vi "PhotoEncoder.vi"(6 "Value":bool, 7 "Array":i16[](array[numeric]), 9 "Numeric 2":dbl, 10 "DigitalInputDevRef":T1, 11 "Numeric":dbl) -> ()   [LabVIEW 2015]
uses:
  <vilib>/Rock Robotics/WPI/DigitalInput/WPI_DigitalInputDevRef.ctl
  <vilib>/Rock Robotics/SystemInterfaces/DIO/FPGA_DIOChannel.ctl
  Wheel Gun Test/Robot Global Data.vi
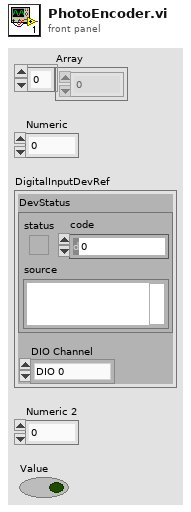
[diagram p1: front panel]
types:
  T1 = typedef "WPI_DigitalInputDevRef.ctl" = cluster{"DevStatus":errorcluster, "DIO Channel":T2}
  T2 = typedef "FPGA_DIOChannel.ctl" = enum8{"DIO 0", "DIO 1", "DIO 2", "DIO 3", "DIO 4", "DIO 5", "DIO 6", "DIO 7", "DIO 8", "DIO 9", "DIO MXP 0", "DIO MXP 1", "DIO MXP 2", "DIO MXP 3", "DIO MXP 4", "DIO MXP 5", "DIO MXP 6", "DIO MXP 7", "DIO MXP 8", "DIO MXP 9", "DIO MXP 10", "DIO MXP 11", "DIO MXP 12", "DIO MXP 13", "DIO MXP 14", "DIO MXP 15", "Invalid"}
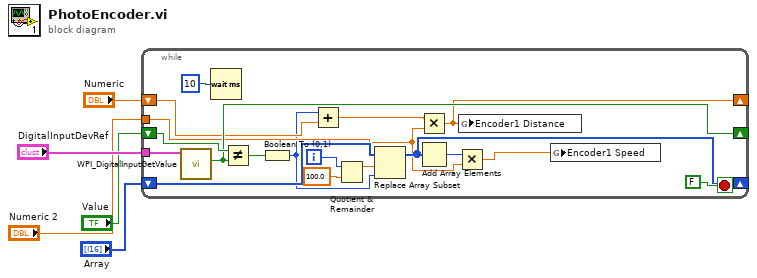
[diagram p0: block diagram]
diagram:
  n1 = while {
    shift-right: [w20] -> _
    shift-left: "Value" -> [w21]
    shift-right: [w8] -> _
    shift-left: "Numeric" -> [w19]
    shift-right: [w17] -> _
    shift-left: "Array" -> [w18]
    tunnel: "Numeric 2" -> [w14]
    tunnel: "DigitalInputDevRef" -> [w9]
    i -> [w12]
    stop <- FALSE stop-if-true
    n2 = call <vilib>:"WPI_DigitalInputGetValue.vi"("DigitalInputDevRef"=w9) -> ("Value"=w20:bool)  [unwired: 8 in, 2 out]
    n3 = Wait (ms)(milliseconds to wait=u32 10) -> ()  [unwired: 1 out]
    n4 = Not Equal?(x=w21, y=w20) -> (x != y?=w16:bool)
    n5 = Boolean To (0,1)(Boolean=w16) -> (0, 1=w10:i16)
    n6 = Add(x=w10, y=w19) -> (x+y=w6:dbl)
    n7 = Quotient & Remainder(x=w12, y=100.0) -> (x-y*floor(x/y)=w11:dbl)  [unwired: 1 out]
    n8 = Replace Array Subset(array=w18, new element=w10, index=w11) -> (w17:i16[])
    n9 = Multiply(x=w6, y=w14) -> (x*y=w8:dbl)
    n10 = Add Array Elements(numeric array=w17) -> (sum=w15:i16)
    n11 = Multiply(x=w15, y=w14) -> (x*y=w7:dbl)
    n12 = global write "Robot Global Data.vi" "Encoder1 Distance"(w8) -> ()
    n13 = global write "Robot Global Data.vi" "Encoder1 Speed"(w7) -> ()
  }
